vi "LWXPS_GatheringConfigurationSet.vi"(0 "XPS Reference IN":refnum<k24>, 5 "Type IN":string[](array[string]), 11 "LabVIEW error IN":errorcluster) -> (4 "XPS Reference OUT":refnum<k24>, 6 "Returned error code":i32, 8 "Type OUT":string[](array[string]), 10 "XPS Error String":string, 15 "LabVIEW error OUT":errorcluster)   [LabVIEW 2014]
uses:
  D:/XPSQ8_LabView_Library/Development/Source/Dll/Newport.XPS.CommandInterface.dll
  Dll/Newport.XPS.CommandInterface.dll
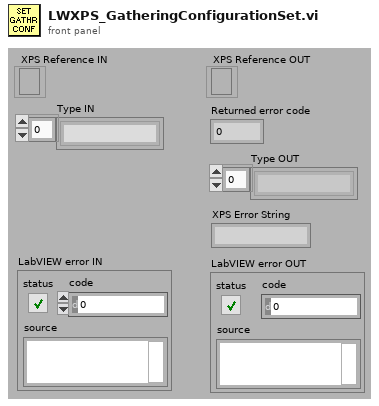
[diagram p1: front panel]
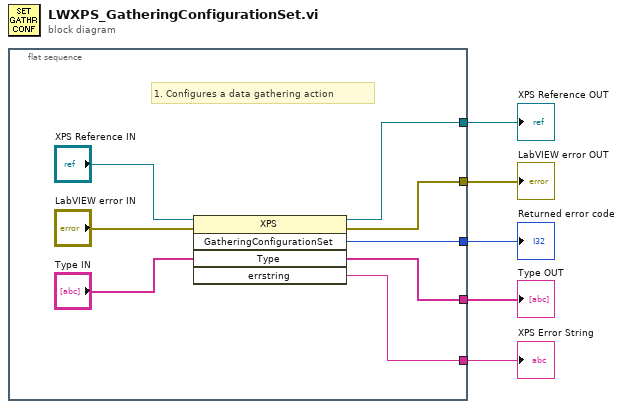
[diagram p0: block diagram]
diagram:
  n1 = flat-sequence {
    tunnel: [w8] -> w5
    tunnel: [w12] -> w4
    tunnel: [w11] -> w3
    tunnel: [w10] -> w2
    tunnel: [w7] -> w1
    frame #0 {
      # "1. Configures a data gathering action"
      n2 = invoke class="XPS" method="GatheringConfigurationSet"(reference="XPS Reference IN", error in="LabVIEW error IN", "Type"="Type IN") -> (reference out=w12:refnum<k24>, error out=w11:errorcluster, "GatheringConfigurationSet"=w10:i32, "Type"=w7:string[], "errstring"=w8:string)  [unwired: 2 in]
    }
  }
  "XPS Error String" <- w5
  "XPS Reference OUT" <- w4
  "LabVIEW error OUT" <- w3
  "Returned error code" <- w2
  "Type OUT" <- w1
